vi "Lecroy_wait_acq-complete.vi"(7 "start (ref)":refnum<vi>, 8 "error in (no error)":errorcluster, 9 "stop (ref)":refnum<vi>, 10 "Timeout (10000 ms)":u32=10000, 11 "VISA resource name":refnum<visa-resource-name>) -> (0 "error out":errorcluster, 2 "Complete":bool, 3 "VISA resource name out":refnum<visa-resource-name>)   [LabVIEW 2010]
doc: "This detect whether previous operation finished in specified time or no."
uses:
  <instrlib>/LeCroy Wave Series/LeCroy Wave Series.lvlib
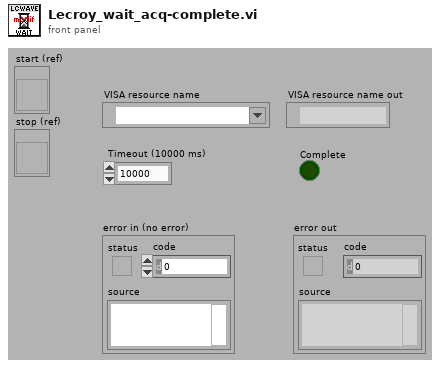
[diagram p1: front panel]
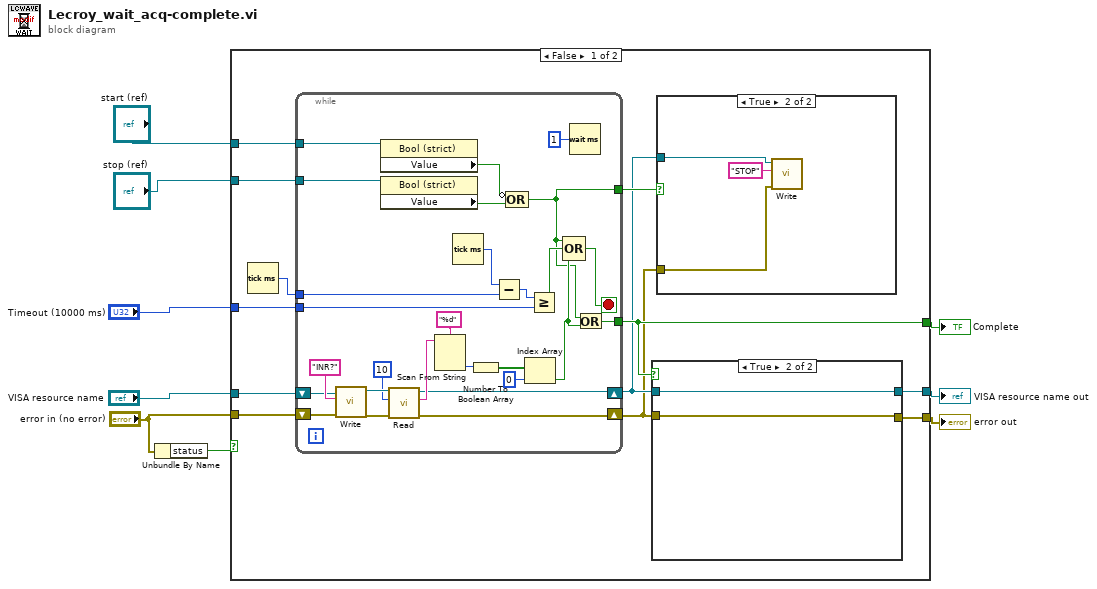
[diagram p0: block diagram]
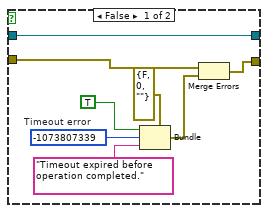
[diagram p3: hidden frame]
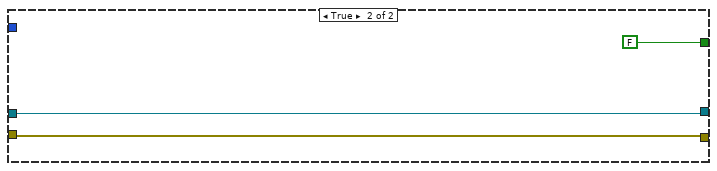
[diagram p4: hidden frame]
diagram:
  n1 = Unbundle By Name("error in (no error)") -> ("status"=w4:bool)
  n2 = case shown="False" w4 {
    tunnel: "VISA resource name" -> [w21 w64]
    tunnel: "Timeout (10000 ms)" -> [w19 _]
    tunnel: [w18 w64] -> w7
    tunnel: [w17 w63] -> w6
    tunnel: "error in (no error)" -> [w16 w63]
    tunnel: [w15 FALSE] -> w3
    tunnel: "start (ref)" -> [w11 _]
    tunnel: "stop (ref)" -> [w10 _]
    frame False {
      n3 = Tick Count (ms)() -> (millisecond timer value=w20:u32)
      n4 = while {
        tunnel: w20 -> [w49]
        tunnel: w19 -> [w47]
        tunnel: [w41] -> w15
        shift-right: [w45] -> w13
        shift-left: w21 -> [w52]
        shift-right: [w44] -> w12
        shift-left: w16 -> [w51]
        tunnel: [w35] -> w14
        tunnel: w11 -> [w39]
        tunnel: w10 -> [w38]
        stop <- w42 stop-if-true
        n5 = call <instrlib>:"Write.vi"("error in (no error)"=w51, "Write Buffer"="INR?" ("write buffer"), "VISA resource name"=w52) -> ("error out"=w60:errorcluster, "VISA resource name out"=w61:refnum<visa-resource-name>)  [unwired: 7 out]
        n6 = property class="Bool (strict)"(reference=w39) -> ("Value"=w37:bool)  [unwired: 1 in, 2 out]
        n7 = property class="Bool (strict)"(reference=w38) -> ("Value"=w36:bool)  [unwired: 1 in, 2 out]
        n8 = call <instrlib>:"Read.vi"("error in (no error)"=w60, "Byte Count"=u32 10 ("byte count"), "VISA resource name"=w61) -> ("error out"=w44:errorcluster, "Read Buffer"=w58:string, "VISA resource name out"=w45:refnum<visa-resource-name>)  [unwired: 6 out]
        n9 = Scan From String(format string="%d", input string=w58) -> (output 1=w55:i32)  [unwired: 2 in, 4 out]
        n10 = Tick Count (ms)() -> (millisecond timer value=w50:u32)
        n11 = Number To Boolean Array(number=w55) -> (Boolean array=w54:bool[])
        n12 = Subtract(x=w50, y=w49) -> (x-y=w48:u32)
        n13 = Compound Arithmetic op=OR(invert w37, w36) -> (w35:bool)
        n14 = Index Array(array=w54, index=0) -> (element=w40:bool)
        n15 = Greater Or Equal?(x=w48, y=w47) -> (x >= y?=w43:bool)
        n16 = Compound Arithmetic op=OR(w35, w43, w40) -> (w42:bool)
        n17 = Wait (ms)(milliseconds to wait=u32 1) -> ()  [unwired: 1 out]
        n18 = Or(x=w35, y=w40) -> (x .or. y?=w41:bool)
      }
      n19 = case shown="True" w15 {
        tunnel: w13 -> [w28 w34]
        tunnel: w12 -> [w26 w33]
        tunnel: [w28 w34] -> w18
        tunnel: [w27 w33] -> w17
        frame False {
          w31 = -1073807339  # Timeout error
          n20 = Bundle(cluster=errorcluster {"status"=FALSE, "code"=0, "source"=""} ("error out"), "status"=TRUE, "code"=w31, "source"="Timeout expired before operation completed." ("Source")) -> (w25:errorcluster)
          n21 = Merge Errors(w26, w25) -> (w27:errorcluster)
        }
        frame True {
        }
      }
      n22 = case shown="True" w14 {
        tunnel: w13 -> [_ w23]
        tunnel: w12 -> [_ w22]
        frame False {
        }
        frame True {
          n23 = call <instrlib>:"Write.vi"("error in (no error)"=w22, "Write Buffer"="STOP", "VISA resource name"=w23) -> ()  [unwired: 9 out]
        }
      }
    }
    frame True {
    }
  }
  "VISA resource name out" <- w7
  "error out" <- w6
  "Complete" <- w3
